vi "Matrix Logarithm.vi"   [LabVIEW 2024, in "NI_AALBase.lvlib"]
doc: "<p>Computes the natural logarithm of a square <strong>Input Matrix</strong>. Wire data to the <strong>Input Matrix</strong> input to determine the polymorphic instance to use or <a href=\"nihelplauncher://docs/csh?context=lvcore_lvhowto_selectingdefaultinstpolyvi\">manually select</a> the instance.</p>"
uses:
  NI_AALBase.lvlib
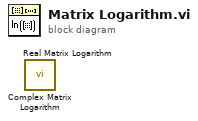
[diagram p0: block diagram]
diagram:
  n1 = call "Complex Matrix Logarithm.vi"() -> ()  [unwired: 2 in, 2 out]
  n2 = call "Real Matrix Logarithm.vi"() -> ()  [unwired: 2 in, 2 out]
